vi "GeoData.vi"() -> ()   [LabVIEW 2017] (continued)
\tGA\tChattooga County\tH1\n30165\t13055\tRome\tGA\tChattooga County\tH1\n30730\t13055\tLyerly\tGA\tChattooga County\tH1\n30731\t13055\tMenlo\tGA\tChattooga County\tH1\n30753\t13055\tTrion\tGA\tChattooga County\tH1\n30747\t13055\tSummerville\tGA\tChattooga County\tH1\n30534\t13057\tDawsonville\tGA\tCherokee County\tH1\n30107\t13057\tBall ground\tGA\tCherokee County\tH1\n30188\t13057\tWoodstock\tGA\tCherokee County\tH1\n30075\t13057\tRoswell\tGA\tCherokee County\tH1\n30102\t13057\tAcworth\tGA\tCherokee County\tH1\n30184\t13057\tWhite\tGA\tCherokee County\tH1\n30101\t13057\tAcworth\tGA\tCherokee County\tH1\n30169\t13057\tCanton\tGA\tCherokee County\tH1\n30151\t13057\tNelson\tGA\tCherokee County\tH1\n30028\t13057\tCumming\tGA\tCherokee County\tH1\n30114\t13057\tCanton\tGA\tCherokee County\tH1\n30139\t13057\tFairmount\tGA\tCherokee County\tH1\n30189\t13057\tWoodstock\tGA\tCherokee County\tH1\n30115\t13057\tCanton\tGA\tCherokee County\tH1\n30183\t13057\tWaleska\tGA\tCherokee County\tH1\n30142\t13057\tHolly springs\tGA\tCherokee County\tH1\n30040\t13057\tCumming\tGA\tCherokee County\tH1\n30066\t13057\tMarietta\tGA\tCherokee County\tH1\n30143\t13057\tJasper\tGA\tCherokee County\tH1\n30004\t13057\tAlpharetta\tGA\tCherokee County\tH1\n30146\t13057\tLebanon\tGA\tCherokee County\tH1\n30604\t13059\tAthens\tGA\tClarke County\tH6\n30603\t13059\tAthens\tGA\tClarke County\tH6\n30607\t13059\tAthens\tGA\tClarke County\tH6\n30683\t13059\tWinterville\tGA\tClarke County\tH6\n30605\t13059\tAthens\tGA\tClarke County\tH6\n30606\t13059\tAthens\tGA\tClarke County\tH6\n30622\t13059\tBogart\tGA\tClarke County\tH6\n30602\t13059\tAthens\tGA\tClarke County\tH6\n30608\t13059\tAthens\tGA\tClarke County\tH6\n30601\t13059\tAthens\tGA\tClarke County\tH6\n30646\t13059\tHull\tGA\tClarke County\tH6\n30609\t13059\tAthens\tGA\tClarke County\tH6\n39854\t13061\tGeorgetown\tGA\tClay County\tH1\n39867\t13061\tMorris\tGA\tClay County\tH1\n39846\t13061\tEdison\tGA\tClay County\tH1\n39824\t13061\tBluffton\tGA\tClay County\tH1\n39823\t13061\tBlakely\tGA\tClay County\tH1\n39836\t13061\tColeman\tGA\tClay County\tH1\n39851\t13061\tFort gaines\tGA\tClay County\tH1\n30236\t13063\tJonesboro\tGA\tClayton County\tH1\n30296\t13063\tRiverdale\tGA\tClayton County\tH1\n30250\t13063\tLovejoy\tGA\tClayton County\tH1\n30273\t13063\tRex\tGA\tClayton County\tH1\n30354\t13063\tAtlanta\tGA\tClayton County\tH1\n30228\t13063\tHampton\tGA\tClayton County\tH1\n30274\t13063\tRiverdale\tGA\tClayton County\tH1\n30294\t13063\tEllenwood\tGA\tClayton County\tH1\n30298\t13063\tForest park\tGA\tClayton County\tH1\n30337\t13063\tAtlanta\tGA\tClayton County\tH1\n30344\t13063\tAtlanta\tGA\tClayton County\tH1\n30238\t13063\tJonesboro\tGA\tClayton County\tH1\n30288\t13063\tConley\tGA\tClayton County\tH1\n30215\t13063\tFayetteville\tGA\tClayton County\tH1\n30260\t13063\tMorrow\tGA\tClayton County\tH1\n30281\t13063\tStockbridge\tGA\tClayton County\tH1\n30297\t13063\tForest park\tGA\tClayton County\tH1\n30320\t13063\tAtlanta\tGA\tClayton County\tH1\n30287\t13063\tMorrow\tGA\tClayton County\tH1\n30349\t13063\tAtlanta\tGA\tClayton County\tH1\n30237\t13063\tJonesboro\tGA\tClayton County\tH1\n31642\t13065\tPearson\tGA\tClinch County\tH1\n31631\t13065\tFargo\tGA\tClinch County\tH1\n31634\t13065\tHomerville\tGA\tClinch County\tH1\n31623\t13065\tArgyle\tGA\tClinch County\tH1\n31635\t13065\tLakeland\tGA\tClinch County\tH1\n31630\t13065\tDu pont\tGA\tClinch County\tH1\n31649\t13065\tStockton\tGA\tClinch County\tH1\n30068\t13067\tMarietta\tGA\tCobb County\tH1\n30144\t13067\tKennesaw\tGA\tCobb County\tH1\n30157\t13067\tDallas\tGA\tCobb County\tH1\n30339\t13067\tAtlanta\tGA\tCobb County\tH1\n30069\t13067\tMarietta\tGA\tCobb County\tH1\n30127\t13067\tPowder springs\tGA\tCobb County\tH1\n30152\t13067\tKennesaw\tGA\tCobb County\tH1\n30188\t13067\tWoodstock\tGA\tCobb County\tH1\n30065\t13067\tMarietta\tGA\tCobb County\tH1\n30075\t13067\tRoswell\tGA\tCobb County\tH1\n30102\t13067\tAcworth\tGA\tCobb County\tH1\n30007\t13067\tMarietta\tGA\tCobb County\tH1\n30008\t13067\tMarietta\tGA\tCobb County\tH1\n30101\t13067\tAcworth\tGA\tCobb County\tH1\n30168\t13067\tAustell\tGA\tCobb County\tH1\n30081\t13067\tSmyrna\tGA\tCobb County\tH1\n30090\t13067\tMarietta\tGA\tCobb County\tH1\n30061\t13067\tMarietta\tGA\tCobb County\tH1\n30080\t13067\tSmyrna\tGA\tCobb County\tH1\n30063\t13067\tMarietta\tGA\tCobb County\tH1\n30060\t13067\tMarietta\tGA\tCobb County\tH1\n30062\t13067\tMarietta\tGA\tCobb County\tH1\n30082\t13067\tSmyrna\tGA\tCobb County\tH1\n30122\t13067\tLithia springs\tGA\tCobb County\tH1\n30126\t13067\tMableton\tGA\tCobb County\tH1\n30160\t13067\tKennesaw\tGA\tCobb County\tH1\n30066\t13067\tMarietta\tGA\tCobb County\tH1\n30067\t13067\tMarietta\tGA\tCobb County\tH1\n31139\t13067\tAtlanta\tGA\tCobb County\tH1\n30006\t13067\tMarietta\tGA\tCobb County\tH1\n30064\t13067\tMarietta\tGA\tCobb County\tH1\n30106\t13067\tAustell\tGA\tCobb County\tH1\n30141\t13067\tHiram\tGA\tCobb County\tH1\n30111\t13067\tClarkdale\tGA\tCobb County\tH1\n30156\t13067\tKennesaw\tGA\tCobb County\tH1\n31532\t13069\tDenton\tGA\tCoffee County\tH1\n31552\t13069\tMillwood\tGA\tCoffee County\tH1\n31624\t13069\tAxson\tGA\tCoffee County\tH1\n31642\t13069\tPearson\tGA\tCoffee County\tH1\n31650\t13069\tWillacoochee\tGA\tCoffee County\tH1\n31519\t13069\tBroxton\tGA\tCoffee County\tH1\n31533\t13069\tDouglas\tGA\tCoffee County\tH1\n31535\t13069\tDouglas\tGA\tCoffee County\tH1\n31567\t13069\tWest green\tGA\tCoffee County\tH1\n31798\t13069\tWray\tGA\tCoffee County\tH1\n31534\t13069\tDouglas\tGA\tCoffee County\tH1\n31554\t13069\tNicholls\tGA\tCoffee County\tH1\n31512\t13069\tAmbrose\tGA\tCoffee County\tH1\n31738\t13071\tCoolidge\tGA\tColquitt County\tH1\n31744\t13071\tDoerun\tGA\tColquitt County\tH1\n31775\t13071\tOmega\tGA\tColquitt County\tH1\n31778\t13071\tPavo\tGA\tColquitt County\tH1\n31773\t13071\tOchlocknee\tGA\tColquitt County\tH1\n31776\t13071\tMoultrie\tGA\tColquitt County\tH1\n31722\t13071\tBerlin\tGA\tColquitt County\tH1\n31788\t13071\tMoultrie\tGA\tColquitt County\tH1\n31784\t13071\tSale city\tGA\tColquitt County\tH1\n31765\t13071\tMeigs\tGA\tColquitt County\tH1\n31768\t13071\tMoultrie\tGA\tColquitt County\tH1\n31753\t13071\tFunston\tGA\tColquitt County\tH1\n31789\t13071\tSumner\tGA\tColquitt County\tH1\n31637\t13071\tLenox\tGA\tColquitt County\tH1\n31771\t13071\tNorman park\tGA\tColquitt County\tH1\n31747\t13071\tEllenton\tGA\tColquitt County\tH1\n31756\t13071\tHartsfield\tGA\tColquitt County\tH1\n30824\t13073\tThomson\tGA\tColumbia County\tH1\n30814\t13073\tHarlem\tGA\tColumbia County\tH1\n30809\t13073\tEvans\tGA\tColumbia County\tH1\n30909\t13073\tAugusta\tGA\tColumbia County\tH1\n30802\t13073\tAppling\tGA\tColumbia County\tH1\n30907\t13073\tAugusta\tGA\tColumbia County\tH1\n30813\t13073\tGrovetown\tGA\tColumbia County\tH1\n30917\t13073\tAugusta\tGA\tColumbia County\tH1\n31647\t13075\tSparks\tGA\tCook County\tH1\n31627\t13075\tCecil\tGA\tCook County\tH1\n31620\t13075\tAdel\tGA\tCook County\tH1\n31632\t13075\tHahira\tGA\tCook County\tH1\n31637\t13075\tLenox\tGA\tCook County\tH1\n30271\t13077\tNewnan\tGA\tCoweta County\tH1\n30265\t13077\tNewnan\tGA\tCoweta County\tH1\n30217\t13077\tFranklin\tGA\tCoweta County\tH1\n30251\t13077\tLuthersville\tGA\tCoweta County\tH1\n30230\t13077\tHogansville\tGA\tCoweta County\tH1\n30289\t13077\tTurin\tGA\tCoweta County\tH1\n30275\t13077\tSargent\tGA\tCoweta County\tH1\n30220\t13077\tGrantville\tGA\tCoweta County\tH1\n30276\t13077\tSenoia\tGA\tCoweta County\tH1\n30268\t13077\tPalmetto\tGA\tCoweta County\tH1\n30277\t13077\tSharpsburg\tGA\tCoweta County\tH1\n30229\t13077\tHaralson\tGA\tCoweta County\tH1\n30259\t13077\tMoreland\tGA\tCoweta County\tH1\n30263\t13077\tNewnan\tGA\tCoweta County\tH1\n30264\t13077\tNewnan\tGA\tCoweta County\tH1\n31016\t13079\tCulloden\tGA\tCrawford County\tH1\n31078\t13079\tRoberta\tGA\tCrawford County\tH1\n31066\t13079\tMusella\tGA\tCrawford County\tH1\n31008\t13079\tByron\tGA\tCrawford County\tH1\n31030\t13079\tFort valley\tGA\tCrawford County\tH1\n31052\t13079\tLizella\tGA\tCrawford County\tH1\n31050\t13079\tKnoxville\tGA\tCrawford County\tH1\n31072\t13081\tPitts\tGA\tCrisp County\tH1\n31092\t13081\tVienna\tGA\tCrisp County\tH1\n31015\t13081\tCordele\tGA\tCrisp County\tH1\n31714\t13081\tAshburn\tGA\tCrisp County\tH1\n31796\t13081\tWarwick\tGA\tCrisp County\tH1\n31079\t13081\tRochelle\tGA\tCrisp County\tH1\n31712\t13081\tArabi\tGA\tCrisp County\tH1\n31010\t13081\tCordele\tGA\tCrisp County\tH1\n30752\t13083\tTrenton\tGA\tDade County\tH1\n30738\t13083\tRising fawn\tGA\tDade County\tH1\n30750\t13083\tLookout mountain\tGA\tDade County\tH1\n30731\t13083\tMenlo\tGA\tDade County\tH1\n30757\t13083\tWildwood\tGA\tDade County\tH1\n30534\t13085\tDawsonville\tGA\tDawson County\tH1\n30536\t13085\tEllijay\tGA\tDawson County\tH1\n30533\t13085\tDahlonega\tGA\tDawson County\tH1\n30028\t13085\tCumming\tGA\tDawson County\tH1\n30143\t13085\tJasper\tGA\tDawson County\tH1\n30148\t13085\tMarble hill\tGA\tDawson County\tH1\n30641\t13085\tGood hope\tGA\tDawson County\tH1\n39834\t13087\tClimax\tGA\tDecatur County\tH1\n39825\t13087\tBrinson\tGA\tDecatur County\tH1\n39817\t13087\tBainbridge\tGA\tDecatur County\tH1\n39815\t13087\tAttapulgus\tGA\tDecatur County\tH1\n39818\t13087\tBainbridge\tGA\tDecatur County\tH1\n39852\t13087\tFowlstown\tGA\tDecatur County\tH1\n39819\t13087\tBainbridge\tGA\tDecatur County\tH1\n31730\t13087\tCamilla\tGA\tDecatur County\tH1\n39837\t13087\tColquitt\tGA\tDecatur County\tH1\n39897\t13087\tWhigham\tGA\tDecatur County\tH1\n30032\t13089\tDecatur\tGA\tDeKalb County\tH1\n30319\t13089\tAtlanta\tGA\tDeKalb County\tH1\n30339\t13089\tAtlanta\tGA\tDeKalb County\tH1\n30031\t13089\tDecatur\tGA\tDeKalb County\tH1\n31107\t13089\tAtlanta\tGA\tDeKalb County\tH1\n30083\t13089\tStone mountain\tGA\tDeKalb County\tH1\n30326\t13089\tAtlanta\tGA\tDeKalb County\tH1\n30341\t13089\tAtlanta\tGA\tDeKalb County\tH1\n30359\t13089\tAtlanta\tGA\tDeKalb County\tH1\n30346\t13089\tAtlanta\tGA\tDeKalb County\tH1\n31119\t13089\tAtlanta\tGA\tDeKalb County\tH1\n30074\t13089\tRedan\tGA\tDeKalb County\tH1\n30033\t13089\tDecatur\tGA\tDeKalb County\tH1\n30035\t13089\tDecatur\tGA\tDeKalb County\tH1\n30039\t13089\tSnellville\tGA\tDeKalb County\tH1\n30316\t13089\tAtlanta\tGA\tDeKalb County\tH1\n30030\t13089\tDecatur\tGA\tDeKalb County\tH1\n30036\t13089\tDecatur\tGA\tDeKalb County\tH1\n30093\t13089\tNorcross\tGA\tDeKalb County\tH1\n31145\t13089\tAtlanta\tGA\tDeKalb County\tH1\n30002\t13089\tAvondale estates\tGA\tDeKalb County\tH1\n30012\t13089\tConyers\tGA\tDeKalb County\tH1\n30079\t13089\tScottdale\tGA\tDeKalb County\tH1\n30087\t13089\tStone mountain\tGA\tDeKalb County\tH1\n30085\t13089\tTucker\tGA\tDeKalb County\tH1\n30294\t13089\tEllenwood\tGA\tDeKalb County\tH1\n30338\t13089\tAtlanta\tGA\tDeKalb County\tH1\n30345\t13089\tAtlanta\tGA\tDeKalb County\tH1\n30360\t13089\tAtlanta\tGA\tDeKalb County\tH1\n31141\t13089\tAtlanta\tGA\tDeKalb County\tH1\n30058\t13089\tLithonia\tGA\tDeKalb County\tH1\n30094\t13089\tConyers\tGA\tDeKalb County\tH1\n30288\t13089\tConley\tGA\tDeKalb County\tH1\n30307\t13089\tAtlanta\tGA\tDeKalb County\tH1\n30329\t13089\tAtlanta\tGA\tDeKalb County\tH1\n30340\t13089\tAtlanta\tGA\tDeKalb County\tH1\n30350\t13089\tAtlanta\tGA\tDeKalb County\tH1\n30366\t13089\tAtlanta\tGA\tDeKalb County\tH1\n30322\t13089\tAtlanta\tGA\tDeKalb County\tH1\n30034\t13089\tDecatur\tGA\tDeKalb County\tH1\n30038\t13089\tLithonia\tGA\tDeKalb County\tH1\n30084\t13089\tTucker\tGA\tDeKalb County\tH1\n30328\t13089\tAtlanta\tGA\tDeKalb County\tH1\n30333\t13089\tAtlanta\tGA\tDeKalb County\tH1\n31146\t13089\tAtlanta\tGA\tDeKalb County\tH1\n30021\t13089\tClarkston\tGA\tDeKalb County\tH1\n30088\t13089\tStone mountain\tGA\tDeKalb County\tH1\n30306\t13089\tAtlanta\tGA\tDeKalb County\tH1\n30315\t13089\tAtlanta\tGA\tDeKalb County\tH1\n30317\t13089\tAtlanta\tGA\tDeKalb County\tH1\n30324\t13089\tAtlanta\tGA\tDeKalb County\tH1\n30037\t13089\tDecatur\tGA\tDeKalb County\tH1\n30072\t13089\tPine lake\tGA\tDeKalb County\tH1\n30086\t13089\tStone mountain\tGA\tDeKalb County\tH1\n30356\t13089\tAtlanta\tGA\tDeKalb County\tH1\n30362\t13089\tAtlanta\tGA\tDeKalb County\tH1\n39901\t13089\tAtlanta\tGA\tDeKalb County\tH1\n31011\t13091\tChauncey\tGA\tDodge County\tH1\n31036\t13091\tHawkinsville\tGA\tDodge County\tH1\n31037\t13091\tMc rae helena\tGA\tDodge County\tH1\n31060\t13091\tMilan\tGA\tDodge County\tH1\n31022\t13091\tDudley\tGA\tDodge County\tH1\n31014\t13091\tCochran\tGA\tDodge County\tH1\n31012\t13091\tChester\tGA\tDodge County\tH1\n31077\t13091\tRhine\tGA\tDodge County\tH1\n31023\t13091\tEastman\tGA\tDodge County\tH1\n31072\t13093\tPitts\tGA\tDooly County\tH1\n31007\t13093\tByromville\tGA\tDooly County\tH1\n31063\t13093\tMontezuma\tGA\tDooly County\tH1\n31092\t13093\tVienna\tGA\tDooly County\tH1\n31015\t13093\tCordele\tGA\tDooly County\tH1\n31071\t13093\tPineview\tGA\tDooly County\tH1\n31091\t13093\tUnadilla\tGA\tDooly County\tH1\n31051\t13093\tLilly\tGA\tDooly County\tH1\n31070\t13093\tPinehurst\tGA\tDooly County\tH1\n31791\t13095\tSylvester\tGA\tDougherty County\tH1\n31702\t13095\tAlbany\tGA\tDougherty County\tH1\n31721\t13095\tAlbany\tGA\tDougherty County\tH1\n39842\t13095\tDawson\tGA\tDougherty County\tH1\n31703\t13095\tAlbany\tGA\tDougherty County\tH1\n31707\t13095\tAlbany\tGA\tDougherty County\tH1\n31701\t13095\tAlbany\tGA\tDougherty County\tH1\n31704\t13095\tAlbany\tGA\tDougherty County\tH1\n31708\t13095\tAlbany\tGA\tDougherty County\tH1\n31763\t13095\tLeesburg\tGA\tDougherty County\tH1\n31706\t13095\tAlbany\tGA\tDougherty County\tH1\n31782\t13095\tPutney\tGA\tDougherty County\tH1\n31705\t13095\tAlbany\tGA\tDougherty County\tH1\n30134\t13097\tDouglasville\tGA\tDouglas County\tH1\n30185\t13097\tWhitesburg\tGA\tDouglas County\tH1\n30154\t13097\tDouglasville\tGA\tDouglas County\tH1\n30127\t13097\tPowder springs\tGA\tDouglas County\tH1\n30187\t13097\tWinston\tGA\tDouglas County\tH1\n30168\t13097\tAustell\tGA\tDouglas County\tH1\n30180\t13097\tVilla rica\tGA\tDouglas County\tH1\n30122\t13097\tLithia springs\tGA\tDouglas County\tH1\n30133\t13097\tDouglasville\tGA\tDouglas County\tH1\n30135\t13097\tDouglasville\tGA\tDouglas County\tH1\n30106\t13097\tAustell\tGA\tDouglas County\tH1\n39841\t13099\tDamascus\tGA\tEarly County\tH1\n39824\t13099\tBluffton\tGA\tEarly County\tH1\n39823\t13099\tBlakely\tGA\tEarly County\tH1\n39845\t13099\tDonalsonville\tGA\tEarly County\tH1\n39861\t13099\tJakin\tGA\tEarly County\tH1\n39832\t13099\tCedar springs\tGA\tEarly County\tH1\n39813\t13099\tArlington\tGA\tEarly County\tH1\n39837\t13099\tColquitt\tGA\tEarly County\tH1\n31636\t13101\tLake park\tGA\tEchols County\tH1\n31631\t13101\tFargo\tGA\tEchols County\tH1\n31648\t13101\tStatenville\tGA\tEchols County\tH1\n31630\t13101\tDu pont\tGA\tEchols County\tH1\n31649\t13101\tStockton\tGA\tEchols County\tH1\n31302\t13103\tBloomingdale\tGA\tEffingham County\tH1\n31312\t13103\tGuyton\tGA\tEffingham County\tH1\n31318\t13103\tMeldrim\tGA\tEffingham County\tH1\n31303\t13103\tClyo\tGA\tEffingham County\tH1\n31307\t13103\tEden\tGA\tEffingham County\tH1\n31407\t13103\tPort wentworth\tGA\tEffingham County\tH1\n30446\t13103\tNewington\tGA\tEffingham County\tH1\n31326\t13103\tRincon\tGA\tEffingham County\tH1\n31329\t13103\tSpringfield\tGA\tEffingham County\tH1\n30635\t13105\tElberton\tGA\tElbert County\tH1\n30634\t13105\tDewy rose\tGA\tElbert County\tH1\n30624\t13105\tBowman\tGA\tElbert County\tH1\n30662\t13105\tRoyston\tGA\tElbert County\tH1\n30457\t13107\tSoperton\tGA\tEmanuel County\tH1\n31002\t13107\tAdrian\tGA\tEmanuel County\tH1\n30448\t13107\tNunez\tGA\tEmanuel County\tH1\n30442\t13107\tMillen\tGA\tEmanuel County\tH1\n30450\t13107\tPortal\tGA\tEmanuel County\tH1\n30436\t13107\tLyons\tGA\tEmanuel County\tH1\n30471\t13107\tTwin city\tGA\tEmanuel County\tH1\n30439\t13107\tMetter\tGA\tEmanuel County\tH1\n31049\t13107\tKite\tGA\tEmanuel County\tH1\n30401\t13107\tSwainsboro\tGA\tEmanuel County\tH1\n30441\t13107\tMidville\tGA\tEmanuel County\tH1\n30474\t13107\tVidalia\tGA\tEmanuel County\tH1\n30464\t13107\tStillmore\tGA\tEmanuel County\tH1\n30425\t13107\tGarfield\tGA\tEmanuel County\tH1\n30477\t13107\tWadley\tGA\tEmanuel County\tH1\n30423\t13109\tDaisy\tGA\tEvans County\tH1\n30420\t13109\tCobbtown\tGA\tEvans County\tH1\n30429\t13109\tHagan\tGA\tEvans County\tH1\n30421\t13109\tCollins\tGA\tEvans County\tH1\n30452\t13109\tRegister\tGA\tEvans County\tH1\n31321\t13109\tPembroke\tGA\tEvans County\tH1\n30453\t13109\tReidsville\tGA\tEvans County\tH1\n30417\t13109\tClaxton\tGA\tEvans County\tH1\n30414\t13109\tBellville\tGA\tEvans County\tH1\n30427\t13109\tGlennville\tGA\tEvans County\tH1\n30541\t13111\tEpworth\tGA\tFannin County\tH1\n30555\t13111\tMc caysville\tGA\tFannin County\tH1\n30572\t13111\tSuches\tGA\tFannin County\tH1\n30559\t13111\tMineral bluff\tGA\tFannin County\tH1\n30560\t13111\tMorganton\tGA\tFannin County\tH1\n30522\t13111\tCherry log\tGA\tFannin County\tH1\n30512\t13111\tBlairsville\tGA\tFannin County\tH1\n30513\t13111\tBlue ridge\tGA\tFannin County\tH1\n30269\t13113\tPeachtree city\tGA\tFayette County\tH1\n30214\t13113\tFayetteville\tGA\tFayette County\tH1\n30213\t13113\tFairburn\tGA\tFayette County\tH1\n30276\t13113\tSenoia\tGA\tFayette County\tH1\n30205\t13113\tBrooks\tGA\tFayette County\tH1\n30238\t13113\tJonesboro\tGA\tFayette County\tH1\n30215\t13113\tFayetteville\tGA\tFayette County\tH1\n31169\t13113\tPeachtree city\tGA\tFayette County\tH1\n30290\t13113\tTyrone\tGA\tFayette County\tH1\n30124\t13115\tCave spring\tGA\tFloyd County\tH1\n30147\t13115\tLindale\tGA\tFloyd County\tH1\n30701\t13115\tCalhoun\tGA\tFloyd County\tH1\n30105\t13115\tArmuchee\tGA\tFloyd County\tH1\n30165\t13115\tRome\tGA\tFloyd County\tH1\n30164\t13115\tRome\tGA\tFloyd County\tH1\n30103\t13115\tAdairsville\tGA\tFloyd County\tH1\n30149\t13115\tMount berry\tGA\tFloyd County\tH1\n30125\t13115\tCedartown\tGA\tFloyd County\tH1\n30733\t13115\tPlainville\tGA\tFloyd County\tH1\n30129\t13115\tCoosa\tGA\tFloyd County\tH1\n30104\t13115\tAragon\tGA\tFloyd County\tH1\n30161\t13115\tRome\tGA\tFloyd County\tH1\n30145\t13115\tKingston\tGA\tFloyd County\tH1\n30173\t13115\tSilver creek\tGA\tFloyd County\tH1\n30172\t13115\tShannon\tGA\tFloyd County\tH1\n30747\t13115\tSummerville\tGA\tFloyd County\tH1\n30162\t13115\tRome\tGA\tFloyd County\tH1\n30534\t13117\tDawsonville\tGA\tForsyth County\tH1\n30107\t13117\tBall ground\tGA\tForsyth County\tH1\n30506\t13117\tGainesville\tGA\tForsyth County\tH1\n30005\t13117\tAlpharetta\tGA\tForsyth County\tH1\n30024\t13117\tSuwanee\tGA\tForsyth County\tH1\n30028\t13117\tCumming\tGA\tForsyth County\tH1\n30041\t13117\tCumming\tGA\tForsyth County\tH1\n30040\t13117\tCumming\tGA\tForsyth County\tH1\n30097\t13117\tDuluth\tGA\tForsyth County\tH1\n30004\t13117\tAlpharetta\tGA\tForsyth County\tH1\n30520\t13119\tCanon\tGA\tFranklin County\tH1\n30557\t13119\tMartin\tGA\tFranklin County\tH1\n30633\t13119\tDanielsville\tGA\tFranklin County\tH1\n30639\t13119\tFranklin springs\tGA\tFranklin County\tH1\n30521\t13119\tCarnesville\tGA\tFranklin County\tH1\n30538\t13119\tEastanollee\tGA\tFranklin County\tH1\n30577\t13119\tToccoa\tGA\tFranklin County\tH1\n30530\t13119\tCommerce\tGA\tFranklin County\tH1\n30516\t13119\tBowersville\tGA\tFranklin County\tH1\n30553\t13119\tLavonia\tGA\tFranklin County\tH1\n30662\t13119\tRoyston\tGA\tFranklin County\tH1\n30076\t13121\tRoswell\tGA\tFulton County\tH1\n30312\t13121\tAtlanta\tGA\tFulton County\tH1\n30319\t13121\tAtlanta\tGA\tFulton County\tH1\n30339\t13121\tAtlanta\tGA\tFulton County\tH1\n30363\t13121\tAtlanta\tGA\tFulton County\tH1\n31131\t13121\tAtlanta\tGA\tFulton County\tH1\n30369\t13121\tAtlanta\tGA\tFulton County\tH1\n30296\t13121\tRiverdale\tGA\tFulton County\tH1\n30318\t13121\tAtlanta\tGA\tFulton County\tH1\n30326\t13121\tAtlanta\tGA\tFulton County\tH1\n30346\t13121\tAtlanta\tGA\tFulton County\tH1\n30358\t13121\tAtlanta\tGA\tFulton County\tH1\n30361\t13121\tAtlanta\tGA\tFulton County\tH1\n30301\t13121\tAtlanta\tGA\tFulton County\tH1\n30380\t13121\tAtlanta\tGA\tFulton County\tH1\n30075\t13121\tRoswell\tGA\tFulton County\tH1\n30214\t13121\tFayetteville\tGA\tFulton County\tH1\n30310\t13121\tAtlanta\tGA\tFulton County\tH1\n30316\t13121\tAtlanta\tGA\tFulton County\tH1\n30314\t13121\tAtlanta\tGA\tFulton County\tH1\n30354\t13121\tAtlanta\tGA\tFulton County\tH1\n30355\t13121\tAtlanta\tGA\tFulton County\tH1\n30325\t13121\tAtlanta\tGA\tFulton County\tH1\n30377\t13121\tAtlanta\tGA\tFulton County\tH1\n30005\t13121\tAlpharetta\tGA\tFulton County\tH1\n30009\t13121\tAlpharetta\tGA\tFulton County\tH1\n30024\t13121\tSuwanee\tGA\tFulton County\tH1\n30213\t13121\tFairburn\tGA\tFulton County\tH1\n30309\t13121\tAtlanta\tGA\tFulton County\tH1\n30334\t13121\tAtlanta\tGA\tFulton County\tH1\n30364\t13121\tAtlanta\tGA\tFulton County\tH1\n31106\t13121\tAtlanta\tGA\tFulton County\tH1\n30077\t13121\tRoswell\tGA\tFulton County\tH1\n30385\t13121\tAtlanta\tGA\tFulton County\tH1\n30343\t13121\tAtlanta\tGA\tFulton County\tH1\n30308\t13121\tAtlanta\tGA\tFulton County\tH1\n30313\t13121\tAtlanta\tGA\tFulton County\tH1\n30337\t13121\tAtlanta\tGA\tFulton County\tH1\n30338\t13121\tAtlanta\tGA\tFulton County\tH1\n30344\t13121\tAtlanta\tGA\tFulton County\tH1\n30360\t13121\tAtlanta\tGA\tFulton County\tH1\n30023\t13121\tAlpharetta\tGA\tFulton County\tH1\n30378\t13121\tAtlanta\tGA\tFulton County\tH1\n30098\t13121\tDuluth\tGA\tFulton County\tH1\n30268\t13121\tPalmetto\tGA\tFulton County\tH1\n30291\t13121\tUnion city\tGA\tFulton County\tH1\n30307\t13121\tAtlanta\tGA\tFulton County\tH1\n30303\t13121\tAtlanta\tGA\tFulton County\tH1\n30311\t13121\tAtlanta\tGA\tFulton County\tH1\n30342\t13121\tAtlanta\tGA\tFulton County\tH1\n30336\t13121\tAtlanta\tGA\tFulton County\tH1\n30350\t13121\tAtlanta\tGA\tFulton County\tH1\n30272\t13121\tRed oak\tGA\tFulton County\tH1\n30302\t13121\tAtlanta\tGA\tFulton County\tH1\n30357\t13121\tAtlanta\tGA\tFulton County\tH1\n31126\t13121\tAtlanta\tGA\tFulton County\tH1\n31150\t13121\tAtlanta\tGA\tFulton County\tH1\n30368\t13121\tAtlanta\tGA\tFulton County\tH1\n30398\t13121\tAtlanta\tGA\tFulton County\tH1\n30022\t13121\tAlpharetta\tGA\tFulton County\tH1\n30097\t13121\tDuluth\tGA\tFulton County\tH1\n30305\t13121\tAtlanta\tGA\tFulton County\tH1\n30327\t13121\tAtlanta\tGA\tFulton County\tH1\n30328\t13121\tAtlanta\tGA\tFulton County\tH1\n30321\t13121\tAtlanta\tGA\tFulton County\tH1\n31136\t13121\tAtlanta\tGA\tFulton County\tH1\n30304\t13121\tAtlanta\tGA\tFulton County\tH1\n30004\t13121\tAlpharetta\tGA\tFulton County\tH1\n30092\t13121\tPeachtree corners\tGA\tFulton County\tH1\n30306\t13121\tAtlanta\tGA\tFulton County\tH1\n30315\t13121\tAtlanta\tGA\tFulton County\tH1\n30317\t13121\tAtlanta\tGA\tFulton County\tH1\n30331\t13121\tAtlanta\tGA\tFulton County\tH1\n30324\t13121\tAtlanta\tGA\tFulton County\tH1\n30349\t13121\tAtlanta\tGA\tFulton County\tH1\n30332\t13121\tAtlanta\tGA\tFulton County\tH1\n31156\t13121\tAtlanta\tGA\tFulton County\tH1\n30396\t13121\tAtlanta\tGA\tFulton County\tH1\n30388\t13121\tAtlanta\tGA\tFulton County\tH1\n30534\t13123\tDawsonville\tGA\tGilmer County\tH1\n30536\t13123\tEllijay\tGA\tGilmer County\tH1\n30705\t13123\tChatsworth\tGA\tGilmer County\tH1\n30522\t13123\tCherry log\tGA\tGilmer County\tH1\n30540\t13123\tEllijay\tGA\tGilmer County\tH1\n30539\t13123\tEast ellijay\tGA\tGilmer County\tH1\n30175\t13123\tTalking rock\tGA\tGilmer County\tH1\n30513\t13123\tBlue ridge\tGA\tGilmer County\tH1\n30810\t13125\tGibson\tGA\tGlascock County\tH1\n30803\t13125\tAvera\tGA\tGlascock County\tH1\n30828\t13125\tWarrenton\tGA\tGlascock County\tH1\n30823\t13125\tStapleton\tGA\tGlascock County\tH1\n30820\t13125\tMitchell\tGA\tGlascock County\tH1\n31543\t13127\tHortense\tGA\tGlynn County\tH1\n31520\t13127\tBrunswick\tGA\tGlynn County\tH1\n31522\t13127\tSaint simons island\tGA\tGlynn County\tH1\n31523\t13127\tBrunswick\tGA\tGlynn County\tH1\n31524\t13127\tBrunswick\tGA\tGlynn County\tH1\n31527\t13127\tJekyll island\tGA\tGlynn County\tH1\n31566\t13127\tWaynesville\tGA\tGlynn County\tH1\n31561\t13127\tSea island\tGA\tGlynn County\tH1\n31521\t13127\tBrunswick\tGA\tGlynn County\tH1\n31525\t13127\tBrunswick\tGA\tGlynn County\tH1\n30701\t13129\tCalhoun\tGA\tGordon County\tH1\n30746\t13129\tSugar valley\tGA\tGordon County\tH1\n30171\t13129\tRydal\tGA\tGordon County\tH1\n30103\t13129\tAdairsville\tGA\tGordon County\tH1\n30703\t13129\tCalhoun\tGA\tGordon County\tH1\n30733\t13129\tPlainville\tGA\tGordon County\tH1\n30139\t13129\tFairmount\tGA\tGordon County\tH1\n30734\t13129\tRanger\tGA\tGordon County\tH1\n30735\t13129\tResaca\tGA\tGordon County\tH1\n30175\t13129\tTalking rock\tGA\tGordon County\tH1\n30721\t13129\tDalton\tGA\tGordon County\tH1\n30732\t13129\tOakman\tGA\tGordon County\tH1\n39834\t13131\tClimax\tGA\tGrady County\tH1\n31779\t13131\tPelham\tGA\tGrady County\tH1\n31773\t13131\tOchlocknee\tGA\tGrady County\tH1\n31792\t13131\tThomasville\tGA\tGrady County\tH1\n39827\t13131\tCairo\tGA\tGrady County\tH1\n39828\t13131\tCairo\tGA\tGrady County\tH1\n31730\t13131\tCamilla\tGA\tGrady County\tH1\n39897\t13131\tWhigham\tGA\tGrady County\tH1\n39829\t13131\tCalvary\tGA\tGrady County\tH1\n30677\t13133\tWatkinsville\tGA\tGreene County\tH1\n30678\t13133\tWhite plains\tGA\tGreene County\tH1\n30665\t13133\tSiloam\tGA\tGreene County\tH1\n30650\t13133\tMadison\tGA\tGreene County\tH1\n30642\t13133\tGreensboro\tGA\tGreene County\tH1\n30631\t13133\tCrawfordville\tGA\tGreene County\tH1\n30669\t13133\tUnion point\tGA\tGreene County\tH1\n30043\t13135\tLawrenceville\tGA\tGwinnett County\tH1\n30078\t13135\tSnellville\tGA\tGwinnett County\tH1\n30518\t13135\tBuford\tGA\tGwinnett County\tH1\n30548\t13135\tHoschton\tGA\tGwinnett County\tH1\n30620\t13135\tBethlehem\tGA\tGwinnett County\tH1\n30010\t13135\tNorcross\tGA\tGwinnett County\tH1\n30039\t13135\tSnellville\tGA\tGwinnett County\tH1\n30515\t13135\tBuford\tGA\tGwinnett County\tH1\n30011\t13135\tAuburn\tGA\tGwinnett County\tH1\n30024\t13135\tSuwanee\tGA\tGwinnett County\tH1\n30047\t13135\tLilburn\tGA\tGwinnett County\tH1\n30093\t13135\tNorcross\tGA\tGwinnett County\tH1\n30012\t13135\tConyers\tGA\tGwinnett County\tH1\n30017\t13135\tGrayson\tGA\tGwinnett County\tH1\n30087\t13135\tStone mountain\tGA\tGwinnett County\tH1\n30360\t13135\tAtlanta\tGA\tGwinnett County\tH1\n30048\t13135\tLilburn\tGA\tGwinnett County\tH1\n30052\t13135\tLoganville\tGA\tGwinnett County\tH1\n30340\t13135\tAtlanta\tGA\tGwinnett County\tH1\n30350\t13135\tAtlanta\tGA\tGwinnett County\tH1\n30517\t13135\tBraselton\tGA\tGwinnett County\tH1\n30680\t13135\tWinder\tGA\tGwinnett County\tH1\n30049\t13135\tLawrenceville\tGA\tGwinnett County\tH1\n30091\t13135\tNorcross\tGA\tGwinnett County\tH1\n30095\t13135\tDuluth\tGA\tGwinnett County\tH1\n30003\t13135\tNorcross\tGA\tGwinnett County\tH1\n30046\t13135\tLawrenceville\tGA\tGwinnett County\tH1\n30071\t13135\tNorcross\tGA\tGwinnett County\tH1\n30084\t13135\tTucker\tGA\tGwinnett County\tH1\n30097\t13135\tDuluth\tGA\tGwinnett County\tH1\n30096\t13135\tDuluth\tGA\tGwinnett County\tH1\n30519\t13135\tBuford\tGA\tGwinnett County\tH1\n30747\t13135\tSummerville\tGA\tGwinnett County\tH1\n30019\t13135\tDacula\tGA\tGwinnett County\tH1\n30045\t13135\tLawrenceville\tGA\tGwinnett County\tH1\n30044\t13135\tLawrenceville\tGA\tGwinnett County\tH1\n30092\t13135\tPeachtree corners\tGA\tGwinnett County\tH1\n30042\t13135\tLawrenceville\tGA\tGwinnett County\tH1\n30099\t13135\tDuluth\tGA\tGwinnett County\tH1\n30511\t13137\tBaldwin\tGA\tHabersham County\tH1\n30523\t13137\tClarkesville\tGA\tHabersham County\tH1\n30510\t13137\tAlto\tGA\tHabersham County\tH1\n30580\t13137\tTurnerville\tGA\tHabersham County\tH1\n30531\t13137\tCornelia\tGA\tHabersham County\tH1\n30577\t13137\tToccoa\tGA\tHabersham County\tH1\n30571\t13137\tSautee nacoochee\tGA\tHabersham County\tH1\n30563\t13137\tMount airy\tGA\tHabersham County\tH1\n30535\t13137\tDemorest\tGA\tHabersham County\tH1\n30518\t13139\tBuford\tGA\tHall County\tH1\n30527\t13139\tClermont\tGA\tHall County\tH1\n30548\t13139\tHoschton\tGA\tHall County\tH1\n30564\t13139\tMurrayville\tGA\tHall County\tH1\n30502\t13139\tChestnut mountain\tGA\tHall County\tH1\n30506\t13139\tGainesville\tGA\tHall County\tH1\n30510\t13139\tAlto\tGA\tHall County\tH1\n30566\t13139\tOakwood\tGA\tHall County\tH1\n30507\t13139\tGainesville\tGA\tHall County\tH1\n30533\t13139\tDahlonega\tGA\tHall County\tH1\n30543\t13139\tGillsville\tGA\tHall County\tH1\n30503\t13139\tGainesville\tGA\tHall County\tH1\n30531\t13139\tCornelia\tGA\tHall County\tH1\n30542\t13139\tFlowery branch\tGA\tHall County\tH1\n30517\t13139\tBraselton\tGA\tHall County\tH1\n30501\t13139\tGainesville\tGA\tHall County\tH1\n30504\t13139\tGainesville\tGA\tHall County\tH1\n30519\t13139\tBuford\tGA\tHall County\tH1\n30528\t13139\tCleveland\tGA\tHall County\tH1\n30575\t13139\tTalmo\tGA\tHall County\tH1\n30554\t13139\tLula\tGA\tHall County\tH1\n30567\t13139\tPendergrass\tGA\tHall County\tH1\n30678\t13141\tWhite plains\tGA\tHancock County\tH1\n31094\t13141\tWarthen\tGA\tHancock County\tH1\n31045\t13141\tJewell\tGA\tHancock County\tH1\n31061\t13141\tMilledgeville\tGA\tHancock County\tH1\n31082\t13141\tSandersville\tGA\tHancock County\tH1\n30820\t13141\tMitchell\tGA\tHancock County\tH1\n31087\t13141\tSparta\tGA\tHancock County\tH1\n30179\t13143\tTemple\tGA\tHaralson County\tH1\n30110\t13143\tBremen\tGA\tHaralson County\tH1\n30113\t13143\tBuchanan\tGA\tHaralson County\tH1\n30176\t13143\tTallapoosa\tGA\tHaralson County\tH1\n30182\t13143\tWaco\tGA\tHaralson County\tH1\n30140\t13143\tFelton\tGA\tHaralson County\tH1\n30153\t13143\tRockmart\tGA\tHaralson County\tH1\n31811\t13145\tHamilton\tGA\tHarris County\tH1\n31807\t13145\tEllerslie\tGA\tHarris County\tH1\n31808\t13145\tFortson\tGA\tHarris County\tH1\n31804\t13145\tCataula\tGA\tHarris County\tH1\n31822\t13145\tPine mountain\tGA\tHarris County\tH1\n31826\t13145\tShiloh\tGA\tHarris County\tH1\n31833\t13145\tWest point\tGA\tHarris County\tH1\n31820\t13145\tMidland\tGA\tHarris County\tH1\n31830\t13145\tWarm springs\tGA\tHarris County\tH1\n31831\t13145\tWaverly hall\tGA\tHarris County\tH1\n31823\t13145\tPine mountain valley\tGA\tHarris County\tH1\n31829\t13145\tUpatoi\tGA\tHarris County\tH1\n30520\t13147\tCanon\tGA\tHart County\tH1\n30635\t13147\tElberton\tGA\tHart County\tH1\n30643\t13147\tHartwell\tGA\tHart County\tH1\n30634\t13147\tDewy rose\tGA\tHart County\tH1\n30624\t13147\tBowman\tGA\tHart County\tH1\n30516\t13147\tBowersville\tGA\tHart County\tH1\n30553\t13147\tLavonia\tGA\tHart County\tH1\n30662\t13147\tRoyston\tGA\tHart County\tH1\n30108\t13149\tBowdon\tGA\tHeard County\tH1\n30217\t13149\tFranklin\tGA\tHeard County\tH1\n30230\t13149\tHogansville\tGA\tHeard County\tH1\n30240\t13149\tLagrange\tGA\tHeard County\tH1\n30170\t13149\tRoopville\tGA\tHeard County\tH1\n30263\t13149\tNewnan\tGA\tHeard County\tH1\n30236\t13151\tJonesboro\tGA\tHenry County\tH1\n30223\t13151\tGriffin\tGA\tHenry County\tH1\n30234\t13151\tJenkinsburg\tGA\tHenry County\tH1\n30273\t13151\tRex\tGA\tHenry County\tH1\n30228\t13151\tHampton\tGA\tHenry County\tH1\n30294\t13151\tEllenwood\tGA\tHenry County\tH1\n30252\t13151\tMcdonough\tGA\tHenry County\tH1\n30253\t13151\tMcdonough\tGA\tHenry County\tH1\n30248\t13151\tLocust grove\tGA\tHenry County\tH1\n30281\t13151\tStockbridge\tGA\tHenry County\tH1\n30233\t13151\tJackson\tGA\tHenry County\tH1\n31025\t13153\tElko\tGA\tHouston County\tH1\n31013\t13153\tClinchfield\tGA\tHouston County\tH1\n31088\t13153\tWarner robins\tGA\tHouston County\tH1\n31036\t13153\tHawkinsville\tGA\tHouston County\tH1\n31069\t13153\tPerry\tGA\tHouston County\tH1\n31005\t13153\tBonaire\tGA\tHouston County\tH1\n31047\t13153\tKathleen\tGA\tHouston County\tH1\n31091\t13153\tUnadilla\tGA\tHouston County\tH1\n31095\t13153\tWarner robins\tGA\tHouston County\tH1\n31008\t13153\tByron\tGA\tHouston County\tH1\n31028\t13153\tCenterville\tGA\tHouston County\tH1\n31030\t13153\tFort valley\tGA\tHouston County\tH1\n31093\t13153\tWarner robins\tGA\tHouston County\tH1\n31098\t13153\tWarner robins\tGA\tHouston County\tH1\n31733\t13155\tChula\tGA\tIrwin County\tH1\n31798\t13155\tWray\tGA\tIrwin County\tH1\n31790\t13155\tSycamore\tGA\tIrwin County\tH1\n31774\t13155\tOcilla\tGA\tIrwin County\tH1\n31512\t13155\tAmbrose\tGA\tIrwin County\tH1\n31750\t13155\tFitzgerald\tGA\tIrwin County\tH1\n31783\t13155\tRebecca\tGA\tIrwin County\tH1\n31769\t13155\tMystic\tGA\tIrwin County\tH1\n31749\t13155\tEnigma\tGA\tIrwin County\tH1\n30548\t13157\tHoschton\tGA\tJackson County\tH1\n30565\t13157\tNicholson\tGA\tJackson County\tH1\n30549\t13157\tJefferson\tGA\tJackson County\tH1\n30529\t13157\tCommerce\tGA\tJackson County\tH1\n30558\t13157\tMaysville\tGA\tJackson County\tH1\n30607\t13157\tAthens\tGA\tJackson County\tH1\n30543\t13157\tGillsville\tGA\tJackson County\tH1\n30622\t13157\tBogart\tGA\tJackson County\tH1\n30517\t13157\tBraselton\tGA\tJackson County\tH1\n30680\t13157\tWinder\tGA\tJackson County\tH1\n30666\t13157\tStatham\tGA\tJackson County\tH1\n30530\t13157\tCommerce\tGA\tJackson County\tH1\n30575\t13157\tTalmo\tGA\tJackson County\tH1\n30567\t13157\tPendergrass\tGA\tJackson County\tH1\n30601\t13157\tAthens\tGA\tJackson County\tH1\n30646\t13157\tHull\tGA\tJackson County\tH1\n30599\t13157\tCommerce\tGA\tJackson County\tH1\n30014\t13159\tCovington\tGA\tJasper County\tH1\n31085\t13159\tShady dale\tGA\tJasper County\tH1\n31024\t13159\tEatonton\tGA\tJasper County\tH1\n30055\t13159\tMansfield\tGA\tJasper County\tH1\n31064\t13159\tMonticello\tGA\tJasper County\tH1\n30056\t13159\tNewborn\tGA\tJasper County\tH1\n31038\t13159\tHillsboro\tGA\tJasper County\tH1\n31532\t13161\tDenton\tGA\tJeff Davis County\tH1\n31539\t13161\tHazlehurst\tGA\tJeff Davis County\tH1\n31519\t13161\tBroxton\tGA\tJeff Davis County\tH1\n31510\t13161\tAlma\tGA\tJeff Davis County\tH1\n30810\t13163\tGibson\tGA\tJefferson County\tH1\n30818\t13163\tMatthews\tGA\tJefferson County\tH1\n30803\t13163\tAvera\tGA\tJefferson County\tH1\n30833\t13163\tWrens\tGA\tJefferson County\tH1\n30434\t13163\tLouisville\tGA\tJefferson County\tH1\n30413\t13163\tBartow\tGA\tJefferson County\tH1\n30816\t13163\tKeysville\tGA\tJefferson County\tH1\n30477\t13163\tWadley\tGA\tJefferson County\tH1\n30823\t13163\tStapleton\tGA\tJefferson County\tH1\n30442\t13165\tMillen\tGA\tJenkins County\tH1\n30455\t13165\tRocky ford\tGA\tJenkins County\tH1\n30456\t13165\tSardis\tGA\tJenkins County\tH1\n30441\t13165\tMidville\tGA\tJenkins County\tH1\n30425\t13165\tGarfield\tGA\tJenkins County\tH1\n30822\t13165\tPerkins\tGA\tJenkins County\tH1\n31002\t13167\tAdrian\tGA\tJohnson County\tH1\n31096\t13167\tWrightsville\tGA\tJohnson County\tH1\n31035\t13167\tHarrison\tGA\tJohnson County\tH1\n31089\t13167\tTennille\tGA\tJohnson County\tH1\n31049\t13167\tKite\tGA\tJohnson County\tH1\n30413\t13167\tBartow\tGA\tJohnson County\tH1\n30477\t13167\tWadley\tGA\tJohnson County\tH1\n31211\t13169\tMacon\tGA\tJones County\tH1\n31033\t13169\tHaddock\tGA\tJones County\tH1\n31031\t13169\tGordon\tGA\tJones County\tH1\n31046\t13169\tJuliette\tGA\tJones County\tH1\n31061\t13169\tMilledgeville\tGA\tJones County\tH1\n31217\t13169\tMacon\tGA\tJones County\tH1\n31032\t13169\tGray\tGA\tJones County\tH1\n31038\t13169\tHillsboro\tGA\tJones County\tH1\n31016\t13171\tCulloden\tGA\tLamar County\tH1\n31097\t13171\tYatesville\tGA\tLamar County\tH1\n30204\t13171\tBarnesville\tGA\tLamar County\tH1\n30295\t13171\tZebulon\tGA\tLamar County\tH1\n30224\t13171\tGriffin\tGA\tLamar County\tH1\n30257\t13171\tMilner\tGA\tLamar County\tH1\n30285\t13171\tThe rock\tGA\tLamar County\tH1\n30233\t13171\tJackson\tGA\tLamar County\tH1\n30256\t13171\tMeansville\tGA\tLamar County\tH1\n31605\t13173\tValdosta\tGA\tLanier County\tH1\n31645\t13173\tRay city\tGA\tLanier County\tH1\n31635\t13173\tLakeland\tGA\tLanier County\tH1\n31639\t13173\tNashville\tGA\tLanier County\tH1\n31641\t13173\tNaylor\tGA\tLanier County\tH1\n31649\t13173\tStockton\tGA\tLanier County\tH1\n31002\t13175\tAdrian\tGA\tLaurens County\tH1\n31096\t13175\tWrightsville\tGA\tLaurens County\tH1\n31011\t13175\tChauncey\tGA\tLaurens County\tH1\n30411\t13175\tAlamo\tGA\tLaurens County\tH1\n31075\t13175\tRentz\tGA\tLaurens County\tH1\n31040\t13175\tDublin\tGA\tLaurens County\tH1\n31021\t13175\tDublin\tGA\tLaurens County\tH1\n31037\t13175\tMc rae helena\tGA\tLaurens County\tH1\n30454\t13175\tRockledge\tGA\tLaurens County\tH1\n31022\t13175\tDudley\tGA\tLaurens County\tH1\n31012\t13175\tChester\tGA\tLaurens County\tH1\n31009\t13175\tCadwell\tGA\tLaurens County\tH1\n30428\t13175\tGlenwood\tGA\tLaurens County\tH1\n31027\t13175\tEast dublin\tGA\tLaurens County\tH1\n31019\t13175\tDexter\tGA\tLaurens County\tH1\n31042\t13175\tIrwinton\tGA\tLaurens County\tH1\n31065\t13175\tMontrose\tGA\tLaurens County\tH1\n31787\t13177\tSmithville\tGA\tLee County\tH1\n31721\t13177\tAlbany\tGA\tLee County\tH1\n39842\t13177\tDawson\tGA\tLee County\tH1\n31707\t13177\tAlbany\tGA\tLee County\tH1\n31701\t13177\tAlbany\tGA\tLee County\tH1\n31763\t13177\tLeesburg\tGA\tLee County\tH1\n31743\t13177\tDe soto\tGA\tLee County\tH1\n31764\t13177\tLeslie\tGA\tLee County\tH1\n31316\t13179\tLudowici\tGA\tLiberty County\tH1\n31309\t13179\tFleming\tGA\tLiberty County\tH1\n31315\t13179\tFort stewart\tGA\tLiberty County\tH1\n31323\t13179\tRiceboro\tGA\tLiberty County\tH1\n31314\t13179\tFort stewart\tGA\tLiberty County\tH1\n31310\t13179\tHinesville\tGA\tLiberty County\tH1\n31320\t13179\tMidway\tGA\tLiberty County\tH1\n31333\t13179\tWalthourville\tGA\tLiberty County\tH1\n31313\t13179\tHinesville\tGA\tLiberty County\tH1\n31301\t13179\tAllenhurst\tGA\tLiberty County\tH1\n30817\t13181\tLincolnton\tGA\tLincoln County\tH1\n30668\t13181\tTignall\tGA\tLincoln County\tH1\n31316\t13183\tLudowici\tGA\tLong County\tH1\n31313\t13183\tHinesville\tGA\tLong County\tH1\n30427\t13183\tGlennville\tGA\tLong County\tH1\n31301\t13183\tAllenhurst\tGA\tLong County\tH1\n31636\t13185\tLake park\tGA\tLowndes County\tH1\n31698\t13185\tValdosta\tGA\tLowndes County\tH1\n31601\t13185\tValdosta\tGA\tLowndes County\tH1\n31699\t13185\tMoody afb\tGA\tLowndes County\tH1\n31605\t13185\tValdosta\tGA\tLowndes County\tH1\n31603\t13185\tValdosta\tGA\tLowndes County\tH1\n31606\t13185\tValdosta\tGA\tLowndes County\tH1\n31632\t13185\tHahira\tGA\tLowndes County\tH1\n31604\t13185\tValdosta\tGA\tLowndes County\tH1\n31645\t13185\tRay city\tGA\tLowndes County\tH1\n31602\t13185\tValdosta\tGA\tLowndes County\tH1\n31635\t13185\tLakeland\tGA\tLowndes County\tH1\n31641\t13185\tNaylor\tGA\tLowndes County\tH1\n30534\t13187\tDawsonville\tGA\tLumpkin County\tH1\n30564\t13187\tMurrayville\tGA\tLumpkin County\tH1\n30533\t13187\tDahlonega\tGA\tLumpkin County\tH1\n30512\t13187\tBlairsville\tGA\tLumpkin County\tH1\n30528\t13187\tCleveland\tGA\tLumpkin County\tH1\n30597\t13187\tDahlonega\tGA\tLumpkin County\tH1\n30824\t13189\tThomson\tGA\tMcDuffie County\tH1\n30814\t13189\tHarlem\tGA\tMcDuffie County\tH1\n30806\t13189\tBoneville\tGA\tMcDuffie County\tH1\n30808\t13189\tDearing\tGA\tMcDuffie County\tH1\n30821\t13189\tNorwood\tGA\tMcDuffie County\tH1\n30802\t13189\tAppling\tGA\tMcDuffie County\tH1\n30828\t13189\tWarrenton\tGA\tMcDuffie County\tH1\n31319\t13191\tMeridian\tGA\tMcIntosh County\tH1\n31323\t13191\tRiceboro\tGA\tMcIntosh County\tH1\n31304\t13191\tCrescent\tGA\tMcIntosh County\tH1\n31331\t13191\tTownsend\tGA\tMcIntosh County\tH1\n31305\t13191\tDarien\tGA\tMcIntosh County\tH1\n31327\t13191\tSapelo island\tGA\tMcIntosh County\tH1\n31711\t13193\tAndersonville\tGA\tMacon County\tH1\n31806\t13193\tEllaville\tGA\tMacon County\tH1\n31076\t13193\tReynolds\tGA\tMacon County\tH1\n31081\t13193\tRupert\tGA\tMacon County\tH1\n31063\t13193\tMontezuma\tGA\tMacon County\tH1\n31069\t13193\tPerry\tGA\tMacon County\tH1\n31068\t13193\tOglethorpe\tGA\tMacon County\tH1\n31041\t13193\tIdeal\tGA\tMacon County\tH1\n31057\t13193\tMarshallville\tGA\tMacon County\tH1\n31091\t13193\tUnadilla\tGA\tMacon County\tH1\n31030\t13193\tFort valley\tGA\tMacon County\tH1\n30565\t13195\tNicholson\tGA\tMadison County\tH1\n30627\t13195\tCarlton\tGA\tMadison County\tH1\n30628\t13195\tColbert\tGA\tMadison County\tH1\n30633\t13195\tDanielsville\tGA\tMadison County\tH1\n30683\t13195\tWinterville\t
